vi "EXDIR-YAML_Inefficient_YAML_to_Tree-like_Dictionary.vi"(10 "YAML in":string) -> (2 "dictionary out":T1, 3 "items":cluster{"key":variant, "value":variant}[](array[cluster]))   [LabVIEW 2016]
uses:
  <userlib>/_OpenG.lib/dictionary/dictionary.llb/Dictionary Object RefNum__ogtk.ctl
  <userlib>/_OpenG.lib/dictionary/dictionary.llb/Dictionary Object RefNum - Enum__ogtk.ctl
  <vilib>/addons/_JKI.lib/Serialization/JSON/JKI JSON Serialization.lvlib
panel:
  out "array":string[](array[string])
  out "YAML in raw":string
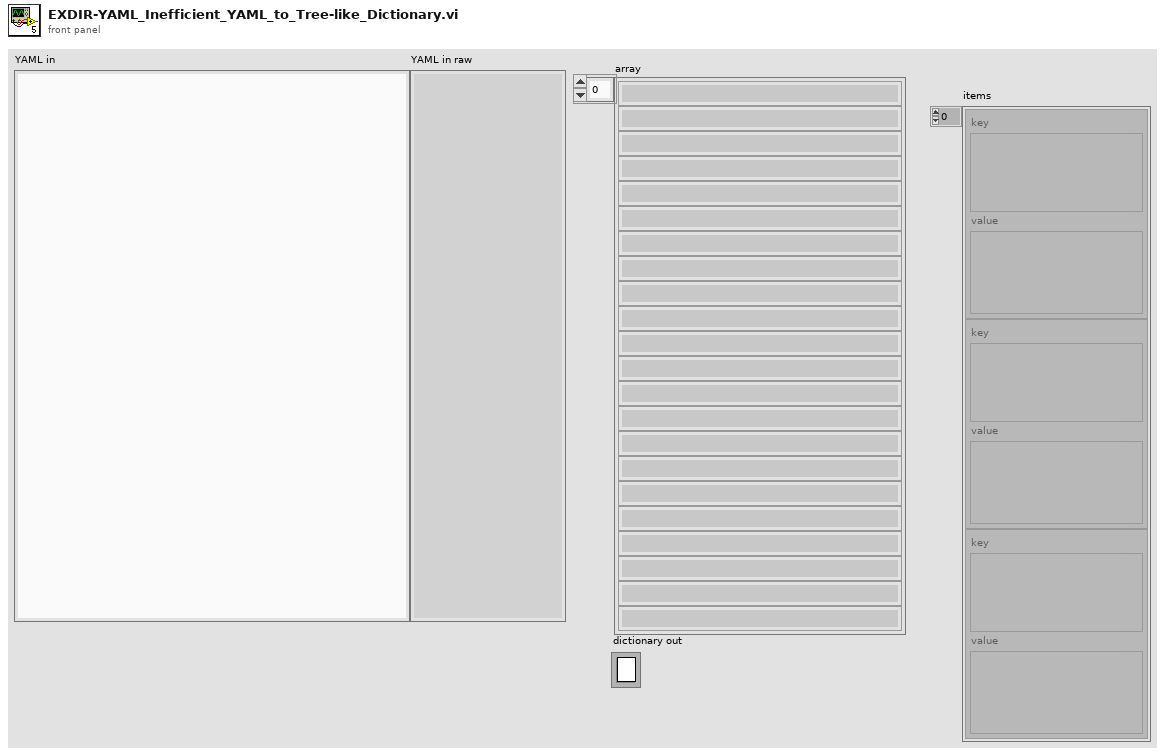
[diagram p1: front panel]
types:
  T1 = typedef "Dictionary Object RefNum__ogtk.ctl" = refnum<k1>
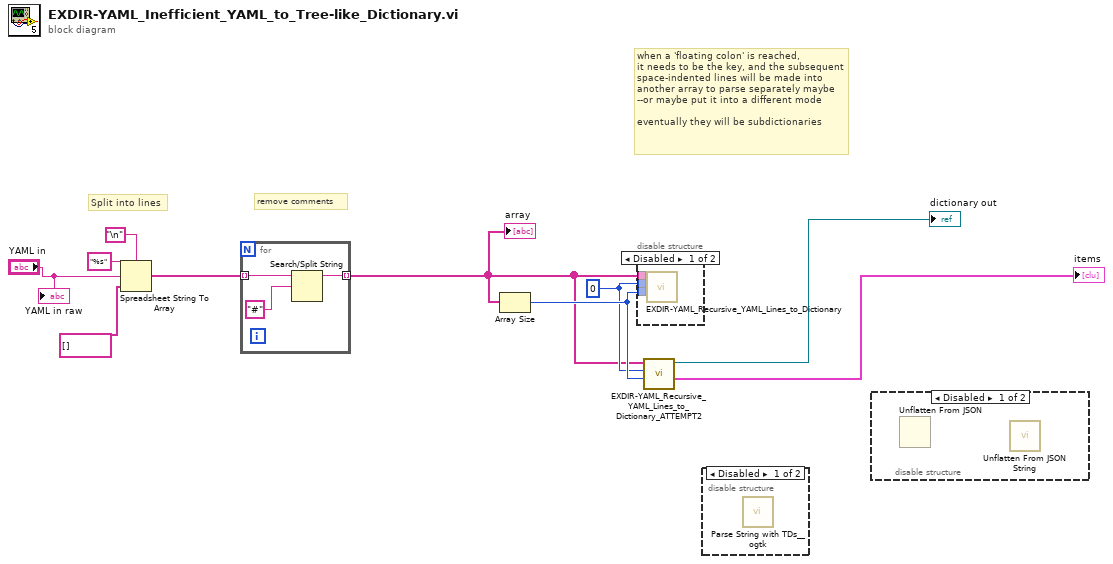
[diagram p0: block diagram]
diagram:
  w5 = 0 ("Start Index")
  # "remove comments"
  # "when a 'floating colon' is reached,\nit needs to be the key, and the subsequent\nspace-indented lines will be made into \nanother array to parse separately maybe\n--or maybe put it into a different mode\n\neventually they will be subdictionaries"
  # "Split into lines"
  n1 = Spreadsheet String To Array(delimiter (Tab)="\n", format string="%s", spreadsheet string="YAML in", array type (2D Dbl)=string[] []) -> (array=w2:string[])
  n2 = for {
    tunnel: w2 -> [w13] mode=indexing
    tunnel: [w11] -> w3 mode=indexing
    n3 = Search/Split String(string=w13, search string/char (-)="#") -> (substring before match=w11:string)  [unwired: 1 in, 2 out]
  }
  "array" <- w3
  n4 = Array Size(array=w3) -> (size(s)=w6:i32)
  n5 = disable-structure shown="Disabled" {
    disable-tunnel: w6 -> [w16 _]
    disable-tunnel: w5 -> [w15 _]
    disable-tunnel: w3 -> [w14 _]
    frame Disabled {
      n6 = call "EXDIR-YAML_Recursive_YAML_Lines_to_Dictionary.vi"("End Index"=w16, "Start Index"=w15, "ENTIRE Array of YAML Lines"=w14) -> ()  [unwired: 6 in, 3 out]
    }
    frame Enabled {
    }
  }
  n7 = call "EXDIR-YAML_Recursive_YAML_Lines_to_Dictionary_ATTEMPT2.vi"("End Index"=w6, "Start Index"=w5, "ENTIRE Array of YAML Lines"=w3) -> ("items"=→"items":cluster{"key":variant, "value":variant}[], "dictionary out"=→"dictionary out":T1)  [unwired: 7 in]
  n8 = disable-structure shown="Disabled" {
    frame Disabled {
      n9 = call <userlib>:"Parse String with TDs__ogtk.vi"() -> ()  [unwired: 9 in, 3 out]
    }
    frame Enabled {
    }
  }
  n10 = disable-structure shown="Disabled" {
    frame Disabled {
      n11 = Unflatten From JSON() -> ()  [unwired: 7 in, 2 out]
      n12 = call <vilib>:"Unflatten From JSON String.vi"() -> ()  [unwired: 10 in, 2 out]
    }
    frame Enabled {
    }
  }
  "YAML in raw" <- "YAML in"
